vi "GetErrors.vi"(0 "XRef":T12, 1 "Generate Strings?":T1, 2 "State In":T5 {"BlockNodeState"."Draw Style" items=["FunctionBlock", "ExpressVI", "Variable", "Elemental I/O", "32x32 Icon", "FunctionBlockCompact"]; "BlockNodeState"."Terminal Data"."Terminal Flags" format="%.0b"}) -> (14 "Errors":T2, 15 "Errors Present?":T1)   [LabVIEW 2017, in "Set DDT Attributes.lvlib" / "Set DDT Properties.xnode"]
uses:
  <vilib>/express/express signal manip/GetorSetDDTAttributes/Set DDT Attributes/Set DDT Properties.xnode
  <vilib>/XNodeSupport/XNodeXNodeRef.ctl
  <vilib>/XNodeSupport/XNodeBool.ctl
  <vilib>/express/express signal manip/GetorSetDDTAttributes/Set DDT Attributes/State.ctl
  <vilib>/BlockNodeSupport/BlockNodeState.ctl
  <vilib>/BlockNodeSupport/TerminalData.ctl
  <vilib>/picture/picture.llb/imagedata.ctl
  <vilib>/express/express signal manip/GetorSetDDTAttributes/Shared VIs/Attributes data.ctl
  <vilib>/express/express signal manip/GetorSetDDTAttributes/Shared VIs/Input.ctl
  <vilib>/express/express signal manip/GetorSetDDTAttributes/Shared VIs/Attributes name.ctl
  <vilib>/XNodeSupport/XNodeError3Array.ctl
  <vilib>/XNodeSupport/XNodeError3.ctl
  <vilib>/XNodeSupport/XNodeString.ctl
  <vilib>/express/express signal manip/GetorSetDDTAttributes/Shared VIs/Global 1.vi
  <vilib>/XNodeSupport/NI_XNodeSupport.lvlib
  <vilib>/express/express signal manip/GetorSetDDTAttributes/Shared VIs/GetSetShared.lvlib
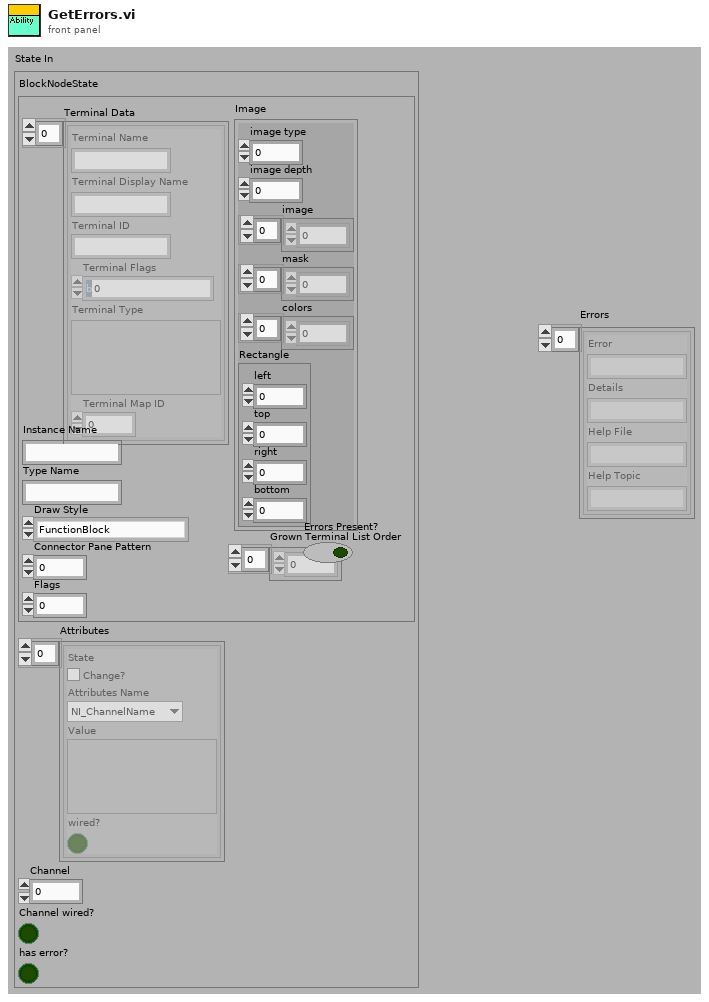
[diagram p1: front panel]
types:
  T1 = typedef "NI_XNodeSupport.lvlib/XNodeBool.ctl" = bool
  T2 = typedef "NI_XNodeSupport.lvlib/XNodeError3Array.ctl" = T3[]
  T3 = typedef "NI_XNodeSupport.lvlib/XNodeError3.ctl" = cluster{"Error":T4, "Details":T4, "Help File":T4, "Help Topic":T4}
  T4 = typedef "NI_XNodeSupport.lvlib/XNodeString.ctl" = string
  T5 = typedef "Set DDT Attributes.lvlib/Set DDT Properties.xnode/State.ctl" = cluster{"BlockNodeState":T6, "Attributes":T9[], "Channel":u32, "Channel wired?":bool, "has error?":bool}
  T6 = typedef "BlockNodeState.ctl" = cluster{"Terminal Data":T7[], "Instance Name":string, "Type Name":string, "Draw Style":i32, "Connector Pane Pattern":i32, "Flags":i32, "Grown Terminal List Order":i32[], "Image":T8}
  T7 = typedef "TerminalData.ctl" = cluster{"Terminal Name":string, "Terminal Display Name":string, "Terminal ID":string, "Terminal Flags":i32, "Terminal Type":variant, "Terminal Map ID":i32}
  T8 = typedef "imagedata.ctl" = cluster{"image type":i32, "image depth":i32, "image":u8[], "mask":u8[], "colors":u32[], "Rectangle":cluster{"left":i16, "top":i16, "right":i16, "bottom":i16}}
  T9 = typedef "GetSetShared.lvlib/Attributes data.ctl" = cluster{"State":T10, "Attributes Name":T11, "Value":variant, "wired?":bool}
  T10 = typedef "GetSetShared.lvlib/Input.ctl" = bool
  T11 = typedef "GetSetShared.lvlib/Attributes name.ctl" = enum16{"NI_ChannelName", "NI_ExpIsRelativeTime", "NI_ExpTimeStamp", "NI_ExpStartTimeStamp", "NI_ExpXDimension", "NI_UnitDescription"}
  T12 = typedef "NI_XNodeSupport.lvlib/XNodeXNodeRef.ctl" = refnum<vi>
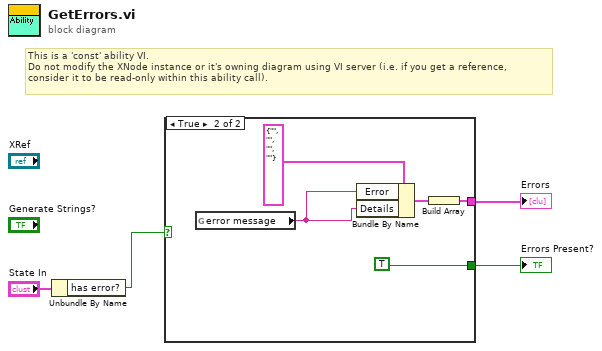
[diagram p0: block diagram]
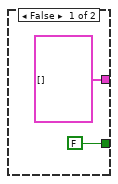
[diagram p2: hidden frame]
diagram:
  # "This is a 'const' ability VI.\nDo not modify the XNode instance or it's owning diagram using VI server (i.e. if you get a reference,\nconsider it to be read-only within this ability call)."
  n1 = Unbundle By Name("State In") -> ("has error?"=w1:bool)
  n2 = case shown="True" w1 {
    tunnel: [T2 [] ("Errors") w7] -> w3
    tunnel: [T1 FALSE ("Errors Present?") T1 TRUE ("Errors Present?")] -> w2
    frame False {
    }
    frame True {
      n3 = global read "Global 1.vi" "error message"() -> (w9:string)
      n4 = Bundle By Name(cluster=T3 {"Error"="", "Details"="", "Help File"="", "Help Topic"=""} ("Error 3"), "Error"=w9, "Details"=w9) -> (w8:T3)
      n5 = Build Array(w8) -> (w7:T3[])
    }
  }
  "Errors" <- w3
  "Errors Present?" <- w2
